vi "Coder.vi"(8 "error in (no error)":errorcluster, 11 "StepMotor in":refnum<class "StepMotor.lvclass">) -> (0 "error out":errorcluster, 3 "StepMotor out":refnum<class "StepMotor.lvclass">)   [LabVIEW 2010, in "StepMotor.lvclass"]
doc: "Кодирование сообщения"
uses:
  StepMotor.lvclass
  StepMotor.lvclass/StepMotor.ctl
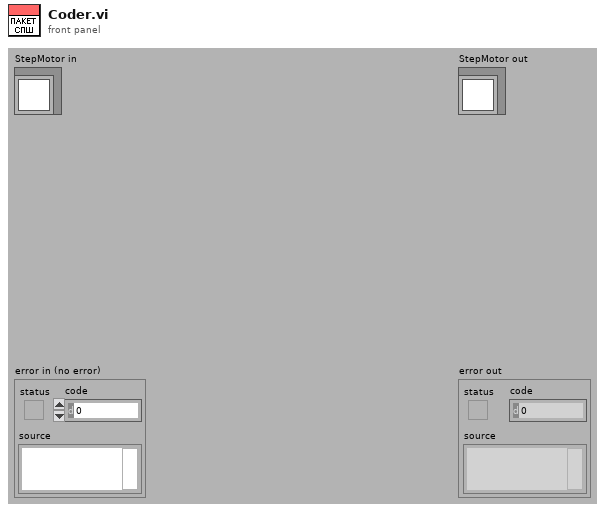
[diagram p1: front panel]
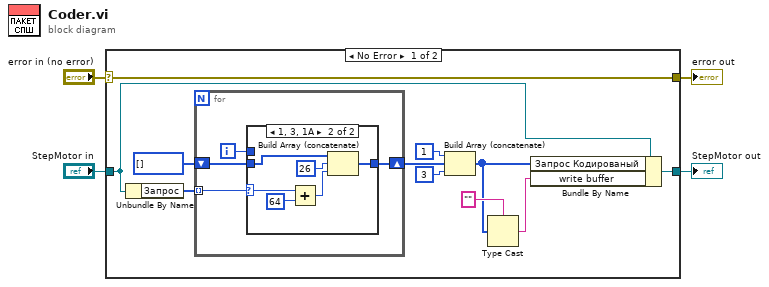
[diagram p0: block diagram]
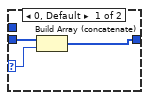
[diagram p2: hidden frame]
diagram:
  n1 = case shown="No Error" "error in (no error)" {
    selector: "error in (no error)" -> [w15 w30]
    tunnel: [w15 w30] -> w3
    tunnel: [w9 w29] -> w1
    tunnel: "StepMotor in" -> [w5 w29]
    frame No Error {
      n2 = Unbundle By Name(w5) -> ("Запрос"=w10:u8[])
      n3 = for {
        tunnel: w10 -> [w19] mode=indexing
        shift-right: [w17] -> w13
        shift-left: u8[] [] ("appended array") -> [w18]
        i -> [w16]
        n4 = case shown="1, 3, 1A" w19 {
          selector: w19 -> [w21 w28]
          tunnel: w18 -> [w22 w24]
          tunnel: [w20 w23] -> w17
          tunnel: w16 -> [_ _]
          frame 0, Default {
            n5 = Build Array (concatenate)(w22, w21) -> (w20:u8[])
          }
          frame 1, 3, 26 {
            n6 = Add(x=w28, y=u8 64 ("Numeric")) -> (x+y=w25:u8)
            n7 = Build Array (concatenate)(w24, u8 26 ("Numeric"), w25) -> (w23:u8[])
          }
        }
      }
      n8 = Build Array (concatenate)(u8 1 ("Numeric"), w13, u8 3 ("Numeric")) -> (w6:u8[])
      n9 = Type Cast(type="" ("write buffer"), x=w6) -> (*(type *) &x=w8:string)
      n10 = Bundle By Name(cluster=w5, "Запрос Кодированый"=w6, "write buffer"=w8) -> (w9:refnum<class "StepMotor.lvclass">)
    }
    frame Error {
    }
  }
  "error out" <- w3
  "StepMotor out" <- w1
